vi "execute_quspin_cmd.vi"(6 "database connection":path, 7 "while loop index":i32, 9 "Controls[]":refnum<vi>[](array[refnum]), 10 "Array":bool[](array[boolean]), 11 "VISA Refnum in":refnum<visa-resource-name>) -> ()   [LabVIEW 2015]
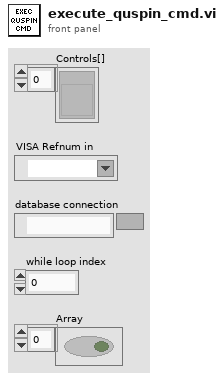
[diagram p1: front panel]
types:
  T1 = typedef "Control 1.ctl" = dbl
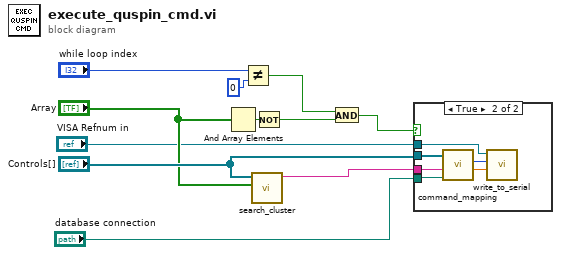
[diagram p0: block diagram]
diagram:
  n1 = And Array Elements(Boolean array="Array") -> (logical AND=w1:bool)
  n2 = Not Equal?(x="while loop index", y=0) -> (x != y?=w8:bool)
  n3 = call "search_cluster.vi"("change?"="Array", "Controls[]"="Controls[]") -> ("Label.Text"=w4:string)  [unwired: 9 in]
  n4 = Not(x=w1) -> (.not. x?=w10:bool)
  n5 = And(x=w8, y=w10) -> (x .and. y?=w9:bool)
  n6 = case shown="True" w9 {
    tunnel: w4 -> [_ w17]
    tunnel: "VISA Refnum in" -> [_ w16]
    tunnel: "Controls[]" -> [_ w13]
    tunnel: "database connection" -> [_ w12]
    frame False {
    }
    frame True {
      n7 = call "command_mapping.vi"("Controls[]"=w13, "cmd in"=w17, "connection information"=w12) -> ("address out"=w15:i16, "value out"=w14:T1)  [unwired: 6 in]
      n8 = call "write_to_serial.vi"("value in"=w14, "address in"=w15, "VISA Refnum in"=w16) -> ()  [unwired: 9 in]
    }
  }
